vi "faraday switch.vi"(2 "cup position":i32=4, 3 "index in":i32, 4 "input fc array":bool[](array[boolean])) -> (0 "index out":i32, 1 "switch cup position?":bool)   [LabVIEW 2016]
doc: "This vi determines if the keithley switch should change or not"
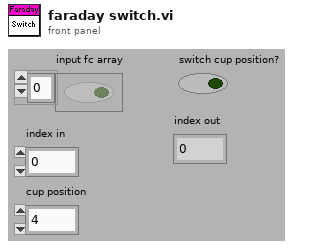
[diagram p1: front panel]
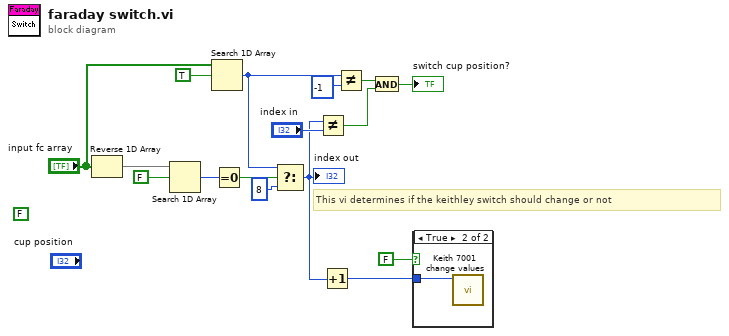
[diagram p0: block diagram]
diagram:
  (unwired) FALSE
  # "This vi determines if the keithley switch should change or not"
  n1 = Reverse 1D Array(array="input fc array") -> (reversed array=w6:bool[])
  n2 = Search 1D Array(1D array=w6, element=FALSE) -> (index of element=w5:i32)  [unwired: 1 out]
  n3 = Search 1D Array(1D array="input fc array", element=TRUE) -> (index of element=w9:i32)  [unwired: 1 out]
  n4 = Equal To 0?(x=w5) -> (x = 0?=w3:bool)
  n5 = Select(t=w9, s=w3, f=u32 8) -> (s? t:f=w2:u32)
  "index out" <- w2
  n6 = Not Equal?(x=w2, y="index in") -> (x != y?=w13:bool)
  n7 = Increment(x=w2) -> (x+1=w14:u32)
  n8 = Not Equal?(x=w9, y=-1) -> (x != y?=w8:bool)
  n9 = And(x=w8, y=w13) -> (x .and. y?=→"switch cup position?":bool)
  n10 = case shown="True" FALSE {
    tunnel: w14 -> [_ w17]
    frame False {
    }
    frame True {
      n11 = call "Keith 7001 change values.vi"("open channel"=w17) -> ()  [unwired: 11 in]
    }
  }
